vi "UIQ_Send(SubVI).vi"(7 "High Priority?":bool, 8 "error in (no error)":errorcluster, 10 "Data":variant, 11 "Command":T1=enum."WaitOnReport") -> (0 "error out":errorcluster)   [LabVIEW 2017, in "MainFrameLib.lvlib"]
uses:
  MainFrameLib.lvlib
  TypeDefs/Command_Enum.ctl
  TypeDefs/QNamesEnum.ctl
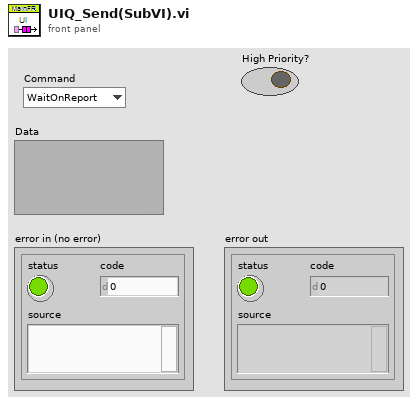
[diagram p1: front panel]
types:
  T1 = typedef "MainFrameLib.lvlib/Command_Enum.ctl" = enum16{"GetSRNotes", "DisplayAEStats", "InWork&Neglected", "RemapAENames", "ClearFolder", "UpdateReportsList", "ExcelReports", "TeamStats", "LoadReport", "WaitOnReport", "RequestReport", "Error", "Idle", "Initialize", "ScreenPop", "ClipboardCopy", "Shutdown"}
  T2 = typedef "MainFrameLib.lvlib/QNamesEnum.ctl" = enum16{"UIQ", "ProcessQ", "CiscoQ", "KCSQ"}
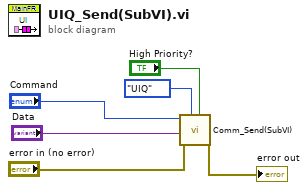
[diagram p0: block diagram]
diagram:
  n1 = call "Comm_Send(SubVI).vi"("High Priority?"="High Priority?", "QueuSelector"=QNamesEnum."UIQ", "Error In"="error in (no error)", "Data"="Data", "Command"="Command") -> ("error out"=→"error out":errorcluster)  [unwired: 6 in]
